vi "Buneman Frequency Estimator PtByPt.vi"(2 "initialize":bool, 3 "sample length":i32=100, 5 "x":dbl format="%0.2f") -> (0 "error":i32, 1 "beta":dbl format="%0.2f")   [LabVIEW 2020, in "NI_PtbyPt.lvlib"]
doc: "Estimates the frequency of a given sine wave of unknown frequency using the Buneman formula."
uses:
  <vilib>/ptbypt/NI_PtbyPt.lvlib
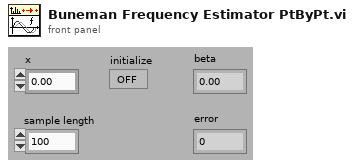
[diagram p1: front panel]
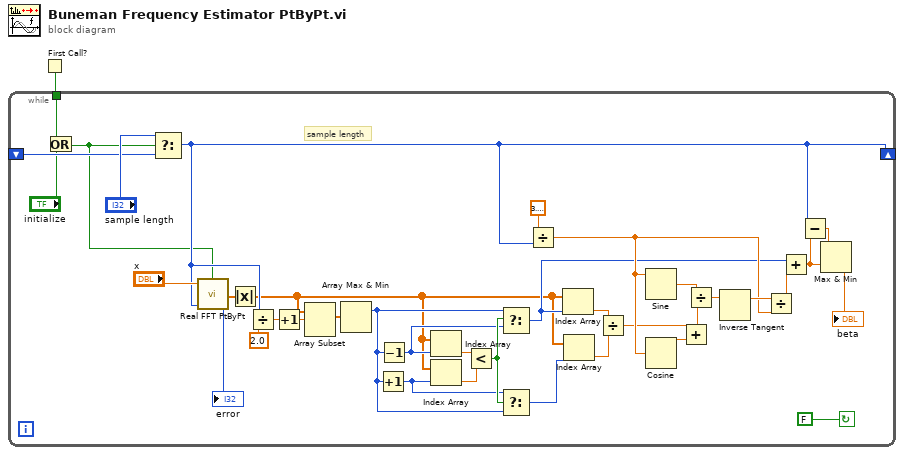
[diagram p0: block diagram]
diagram:
  n1 = First Call?() -> (First Call?: T/F=w1:bool)
  n2 = while {
    tunnel: w1 -> [w5]
    shift-left: _ -> [w19]
    shift-right: [w10] -> _
    stop <- FALSE continue-if-true
    # "sample length"
    n3 = Or(x=w5, y="initialize") -> (x .or. y?=w3:bool)
    n4 = Select(t="sample length", s=w3, f=w19) -> (s? t:f=w10:i32)
    n5 = call <vilib>:"Real FFT PtByPt.vi"("initialize"=w3, "sample length"=w10, "x"="x") -> ("error"=→"error":i32, "FFT{X}"=w38:cdb[])  [unwired: 1 in]
    n6 = Absolute Value(x=w38) -> (abs(x)=w8:dbl[])
    n7 = Divide(x=w10, y=2.0) -> (x/y=w11:dbl)
    n8 = Increment(x=w11) -> (x+1=w9:dbl)
    n9 = Array Subset(array=w8, length=w9) -> (w7:dbl[])  [unwired: 1 in]
    n10 = Array Max & Min(array=w7) -> (max index (indices)=w16:i32)  [unwired: 3 out]
    n11 = Increment(x=w16) -> (x+1=w14:i32)
    n12 = Decrement(x=w16) -> (x-1=w23:i32)
    n13 = Index Array(array=w8, index=w23) -> (element=w36:dbl)
    n14 = Index Array(array=w8, index=w14) -> (element=w37:dbl)
    n15 = Less?(x=w36, y=w37) -> (x < y?=w24:bool)
    n16 = Select(t=w16, s=w24, f=w23) -> (s? t:f=w15:i32)
    n17 = Select(t=w14, s=w24, f=w16) -> (s? t:f=w13:i32)
    n18 = Divide(x=3.141592653589793, y=w10) -> (x/y=w33:dbl)
    n19 = Index Array(array=w8, index=w15) -> (element=w18:dbl)
    n20 = Index Array(array=w8, index=w13) -> (element=w17:dbl)
    n21 = Divide(x=w18, y=w17) -> (x/y=w28:dbl)
    n22 = Sine(x=w33) -> (sin(x)=w30:dbl)
    n23 = Cosine(x=w33) -> (cos(x)=w29:dbl)
    n24 = Add(x=w28, y=w29) -> (x+y=w31:dbl)
    n25 = Divide(x=w30, y=w31) -> (x/y=w32:dbl)
    n26 = Inverse Tangent(1:w32) -> (0:w34:dbl)
    n27 = Divide(x=w34, y=w33) -> (x/y=w35:dbl)
    n28 = Add(x=w15, y=w35) -> (x+y=w26:dbl)
    n29 = Subtract(x=w10, y=w26) -> (x-y=w25:dbl)
    n30 = Max & Min(x=w25, y=w26) -> (min(x,y)=→"beta":dbl)  [unwired: 1 out]
  }
